vi "Console GUI (Read and Write).vi"() -> ()   [LabVIEW 2017, in "Communications Console Library.lvlib"]
uses:
  Communications Console Library.lvlib
  Typedefs/Console GUI-Program State--Enum.ctl
  <vilib>/event_ctls.llb/eventvkey.ctl
  Communications/Typedefs/Functional Global Variable Action--Enum.ctl
  Communications/Communications Library.lvlib
panel:
  out "Sending":bool
  out "Receiving":bool
  in  "User Input":string
  out "Console Text":string
  # "Command to Send"
  # ">"
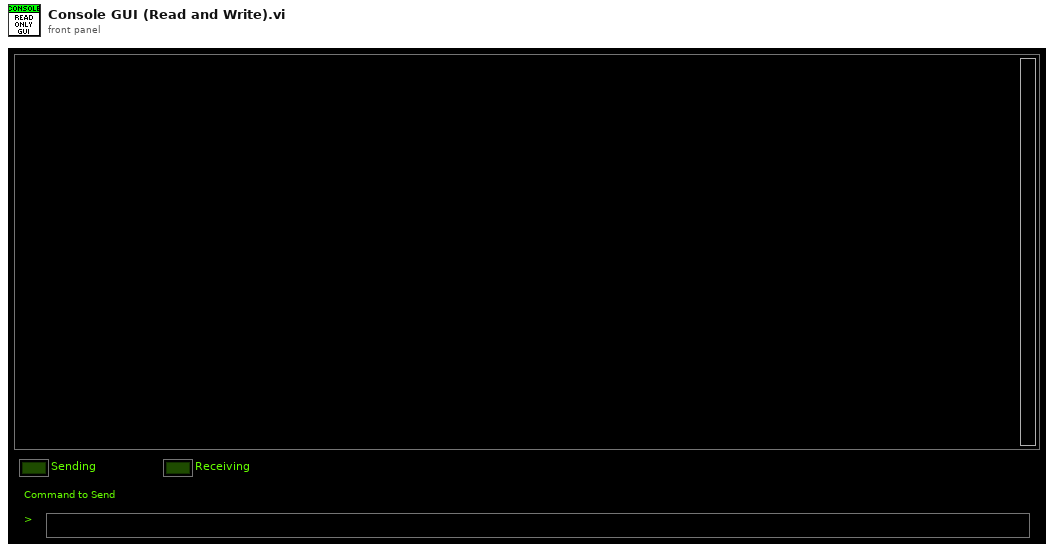
[diagram p1: front panel]
types:
  T1 = typedef "Communications Console Library.lvlib/Console GUI-Program State--Enum.ctl" = enum16{"Load Configuration", "Send Message", "Wait", "Update GUI", "Read TCP Log File"}
  T2 = typedef "eventvkey.ctl" = enum16{"ASCII", "Enter", "Return", "Shift", "Ctrl", "Alt", "Cmd", "Opt", "Caps", "NumLock", "Clear", "Break", "Up", "Down", "Left", "Right", "Insert", "Delete", "Home", "End", "PageUp", "PageDown", "Escape", "Help", "Pause", "ScrollLock", "F1", "F2", "F3", "F4", "F5", "F6", "F7", "F8", "F9", "F10", "F11", "F12", "F13", "F14", "F15", "F16", "F17", "F18", "F19", "F20", "F21", "F22", "F23", "F24", "Play", "VolumeUp", "VolumeDown", "Mute", "Two Byte Char"}
  T3 = typedef "Communications Library.lvlib/Functional Global Variable Action--Enum.ctl" = enum16{"Initialise", "Write Module Config", "Write Carrier Config", "Read"}
  T4 = typedef "Communications Library.lvlib/DTACQ Module Carrier Configuration--Cluster.ctl" = cluster{"Name":string, "IP":string, "Control Port":i32, "Timeout (ms)":i32, "Continuous Capture Port (Multiplexed)":i32, "Start HIL Shot Port":i32, "AWG Upload Port (Multiplexed)":i32, "Download Captured Data Port (Multiplexed)":i32, "Module Slots":i32, "Module Configurations":T5[]}
  T5 = typedef "Communications Library.lvlib/DTACQ Module Configuration--Cluster.ctl" = cluster{"Name":string, "Position":string, "Module Type":T6, "Control Port":i32, "Timeout (ms)":i32, "Channels":i32}
  T6 = typedef "Communications Library.lvlib/DTACQ Device Type--Enum.ctl" = enum16{"Carrier", "Analog In Module", "Analog Out Module", "Generic Module"}
  T7 = typedef "Communications Library.lvlib/DTACQ Connection Data--Cluster.ctl" = cluster{"Description":string, "Address":string, "Port":u16, "timeout (ms)":i32, "Termination Character":string, "TCP Connection Reference":refnum<k5>, "Open Connection":bool}
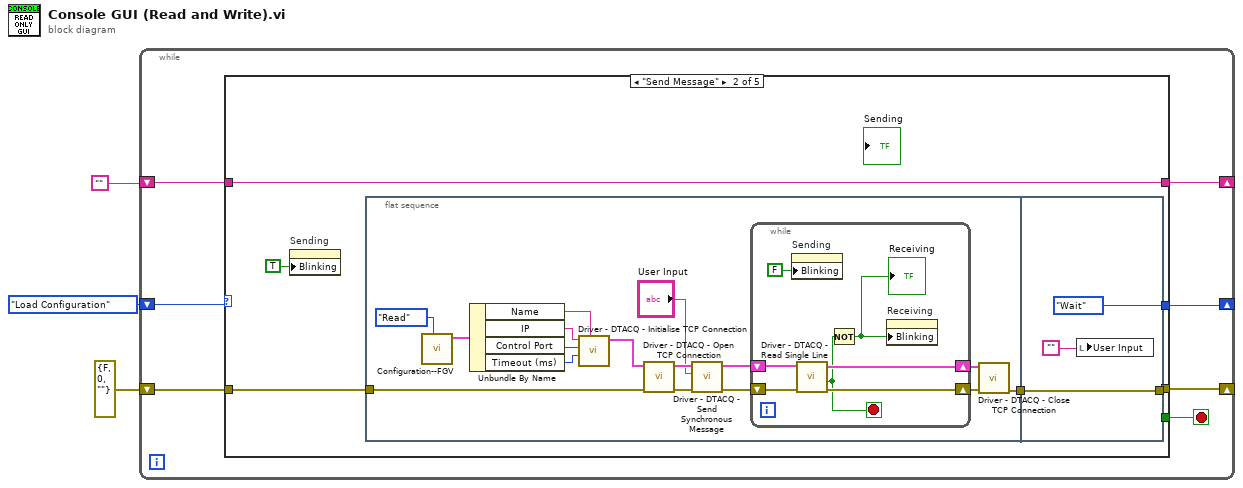
[diagram p0: block diagram]
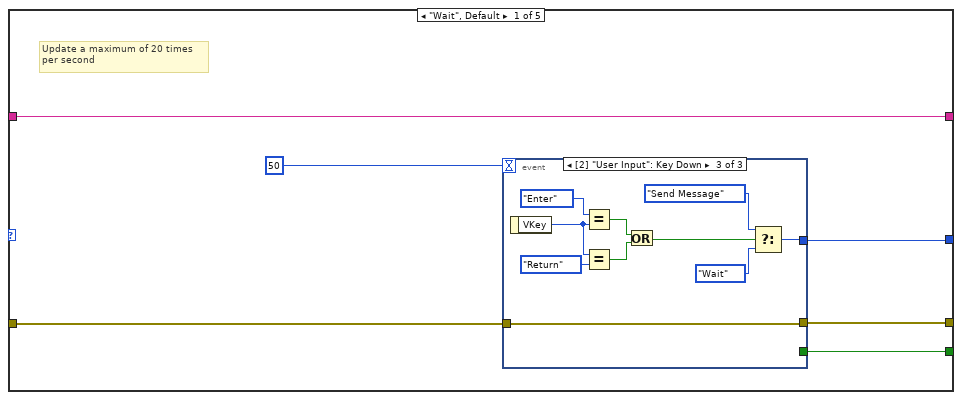
[diagram p2: hidden frame]
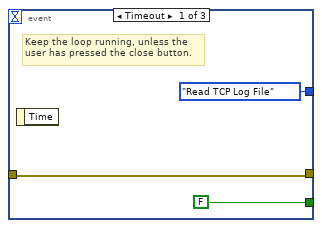
[diagram p3: hidden frame]
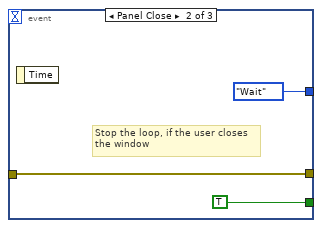
[diagram p4: hidden frame]
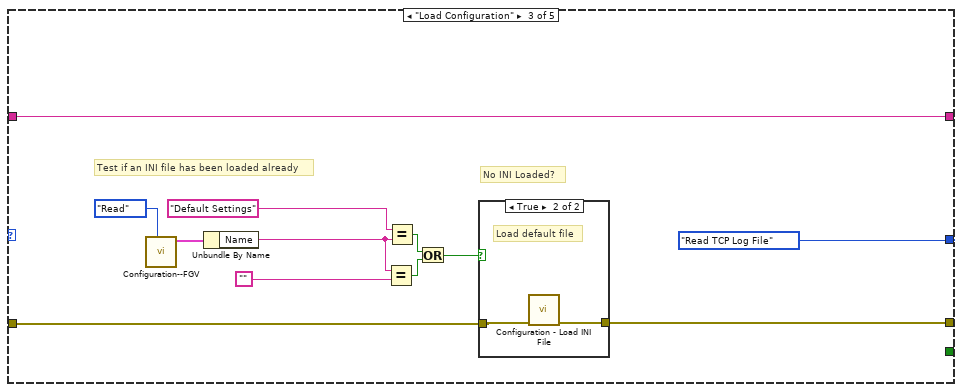
[diagram p5: hidden frame]
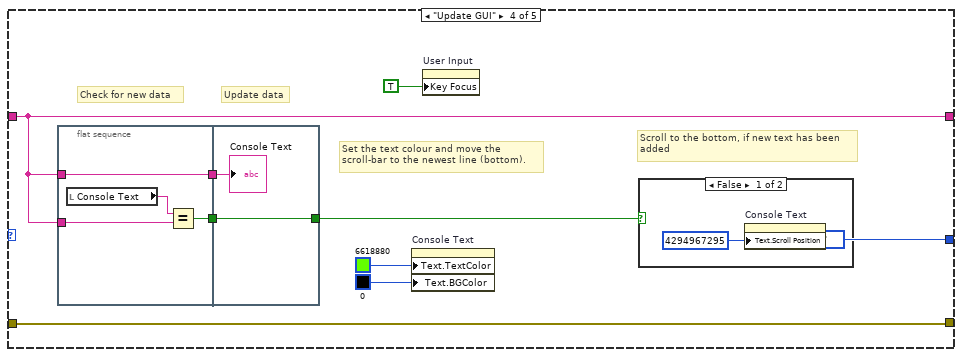
[diagram p7: hidden frame]
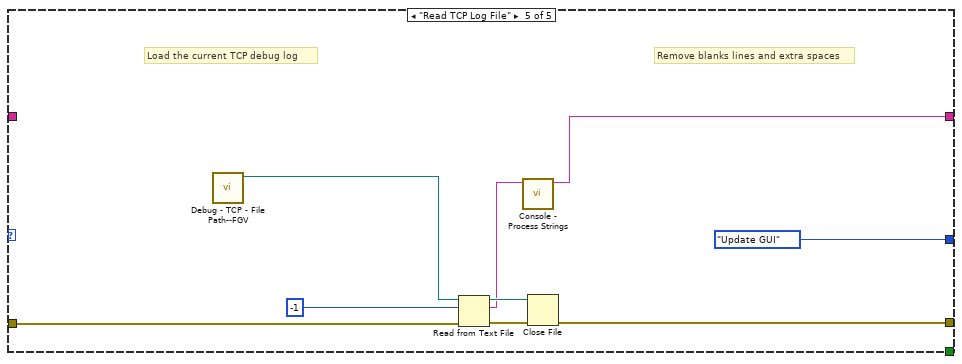
[diagram p9: hidden frame]
diagram:
  n1 = while {
    shift-right: [w10] -> _
    shift-left: "" -> [w9]
    shift-right: [w7] -> _
    shift-left: Console_GUI-Program_State--Enum."Load Configuration" ("Console GUI State") -> [w8]
    shift-right: [w5] -> _
    shift-left: errorcluster {"status"=FALSE, "code"=0, "source"=""} ("error out") -> [w6]
    stop <- w4 stop-if-true
    n2 = case shown="\"Send Message\"" w8 {
      tunnel: [w16 w38 w75 w80 w95] -> w10
      tunnel: w9 -> [w16 w38 w75 w80 _]
      tunnel: [w11 Console_GUI-Program_State--Enum."Wait" ("Console GUI State") Console_GUI-Program_State--Enum."Read TCP Log File" ("Console GUI State") Console_GUI-Program_State--Enum."Wait" ("Console GUI State") Console_GUI-Program_State--Enum."Update GUI" ("Console GUI State")] -> w7
      tunnel: w6 -> [w14 w36 w67 w84 w99]
      tunnel: [w13 w34 w66 w84 w98] -> w5
      tunnel: [w12 _ _ _ _] -> w4
      frame "Wait", Default {
        # "Update a maximum of 20 times\nper second"
        n3 = event shown="[2] \"User Input\": Key Down" {
          selector: _ -> [_ _ _]
          dyn-events: _ -> [_ _ _]
          timeout: 50 -> [_ _ _]
          tunnel: w14 -> [w19 w22 w27]
          tunnel: [w19 w22 w27] -> w13
          tunnel: [FALSE TRUE _] -> w12
          tunnel: [Console_GUI-Program_State--Enum."Read TCP Log File" ("Console GUI State") Console_GUI-Program_State--Enum."Wait" ("Console GUI State") w24] -> w11
          event Timeout {
            # "Keep the loop running, unless the\nuser has pressed the close button."
            n4 = event-data() -> ()  [unwired: 1 in, 1 out]
          }
          event Panel Close {
            # "Stop the loop, if the user closes\nthe window"
            n5 = event-data() -> ()  [unwired: 1 in, 1 out]
          }
          event "User Input": Key Down {
            n6 = event-data() -> ("VKey"=w30:T2)  [unwired: 1 in]
            n7 = Equal?(x=eventvkey."Enter" ("VKey"), y=w30) -> (x = y?=w28:bool)
            n8 = Equal?(x=w30, y=eventvkey."Return" ("VKey")) -> (x = y?=w29:bool)
            n9 = Or(x=w28, y=w29) -> (x .or. y?=w25:bool)
            n10 = Select(t=Console_GUI-Program_State--Enum."Send Message" ("Console GUI State"), s=w25, f=Console_GUI-Program_State--Enum."Wait") -> (s? t:f=w24:T1)
          }
        }
      }
      frame "Send Message" {
        n11 = property on="Sending" class="Bool (strict)"("Blinking"=TRUE) -> ()  [unwired: 2 in, 2 out]
        n12 = flat-sequence {
          tunnel: w36 -> [w48]
          tunnel: [w47] -> w35
          tunnel: [w62] -> w34
          tunnel: w35 -> [w62]
          frame #0 {
            n13 = call "Configuration--FGV.vi"("Functional Global Action"=Functional_Global_Variable_Action--Enum."Read") -> ("Carrier Configuration Out"=w46:T4)  [unwired: 9 in, 1 out]
            n14 = Unbundle By Name(w46) -> ("Name"=w52:string, "IP"=w51:string, "Control Port"=w50:i32, "Timeout (ms)"=w49:i32)
            n15 = call "Driver - DTACQ - Initialise TCP Connection.vi"("Description"=w52, "timeout (ms)"=w49, "Port"=w50, "Address"=w51) -> ("DTACQ Connection Data Out"=w53:T7)  [unwired: 7 in]
            n16 = call "Driver - DTACQ - Open TCP Connection.vi"("error in"=w48, "DTACQ Connection Data In"=w53) -> ("error out"=w45:errorcluster, "DTACQ Connection Data Out"=w44:T7)  [unwired: 8 in]
            n17 = call "Driver - DTACQ - Send Synchronous Message.vi"("error in"=w45, "Message to Send"="User Input", "DTACQ Connection Data In"=w44) -> ("error out"=w42:errorcluster, "DTACQ Connection Data Out"=w43:T7)  [unwired: 5 in, 2 out]
            n18 = while {
              shift-right: [w58] -> w40
              shift-left: w43 -> [w61]
              shift-right: [w59] -> w41
              shift-left: w42 -> [w60]
              stop <- w57 stop-if-true
              n19 = property on="Sending" class="Bool (strict)"("Blinking"=FALSE) -> ()  [unwired: 2 in, 2 out]
              n20 = call "Driver - DTACQ - Read Single Line.vi"("error in"=w60, "DTACQ Connection Data In"=w61) -> ("error out"=w59:errorcluster, "Timed Out"=w57:bool, "DTACQ Connection Data Out"=w58:T7)  [unwired: 6 in, 1 out]
              n21 = Not(x=w57) -> (.not. x?=w56:bool)
              "Receiving" <- w56
              n22 = property on="Receiving" class="Bool (strict)"("Blinking"=w56) -> ()  [unwired: 2 in, 2 out]
            }
            n23 = call "Driver - DTACQ - Close TCP Connection.vi"("error in"=w41, "DTACQ Connection Data In"=w40) -> ("error out"=w47:errorcluster)  [unwired: 8 in, 1 out]
          }
          frame #1 {
            n24 = local write "User Input"("") -> ()
          }
        }
      }
      frame "Load Configuration" {
        # "No INI Loaded?"
        # "Test if an INI file has been loaded already"
        n25 = call "Configuration--FGV.vi"("Functional Global Action"=Functional_Global_Variable_Action--Enum."Read") -> ("Carrier Configuration Out"=w73:T4)  [unwired: 9 in, 1 out]
        n26 = Unbundle By Name(w73) -> ("Name"=w72:string)
        n27 = Equal?(x=w72, y="") -> (x = y?=w69:bool)
        n28 = Equal?(x="Default Settings" ("Name"), y=w72) -> (x = y?=w68:bool)
        n29 = Or(x=w68, y=w69) -> (x .or. y?=w65:bool)
        n30 = case shown="True" w65 {
          tunnel: w67 -> [w76 w78]
          tunnel: [w76 w77] -> w66
          frame False {
            # "INI already loaded,\ndo nothing."
          }
          frame True {
            # "Load default file"
            n31 = call "Configuration - Load INI File.vi"("error in"=w78) -> ("error out"=w77:errorcluster)  [unwired: 9 in, 1 out]
          }
        }
      }
      frame "Update GUI" {
        # "Check for new data"
        # "Scroll to the bottom, if new text has been\nadded"
        # "Update data"
        # "Set the text colour and move the \nscroll-bar to the newest line (bottom)."
        n32 = flat-sequence {
          tunnel: w80 -> [w91]
          tunnel: [w89] -> w82
          tunnel: w80 -> [w88]
          tunnel: [w88] -> w81
          tunnel: [w93] -> w79
          tunnel: w82 -> [w93]
          tunnel: w81 -> [w92]
          frame #0 {
            n33 = local read "Console Text"() -> (w90:string)
            n34 = Equal?(x=w90, y=w91) -> (x = y?=w89:bool)
          }
          frame #1 {
            "Console Text" <- w92
          }
        }
        n35 = property on="Console Text" class="Str"("Text.TextColor"=u32 6618880, "Text.BGColor"=u32 0) -> ()  [unwired: 2 in, 2 out]
        n36 = property on="User Input" class="Str"("Key Focus"=TRUE) -> ()  [unwired: 2 in, 2 out]
        n37 = case shown="False" w79 {
          frame False {
            n38 = property on="Console Text" class="Str"("Text.Scroll Position"=u32 4294967295) -> ()  [unwired: 2 in, 2 out]
          }
          frame True {
          }
        }
      }
      frame "Read TCP Log File" {
        # "Remove blanks lines and extra spaces"
        # "Load the current TCP debug log"
        n39 = call "Debug - TCP - File Path--FGV.vi"() -> ("Debug Pathname"=w96:path)  [unwired: 11 in]
        n40 = Read from Text File(file (use dialog)=w96, count=-1, error in=w99) -> (refnum out=w102:refnum<file>, text=w100:string, error out=w101:errorcluster)  [unwired: 1 in, 1 out]
        n41 = call "Console - Process Strings.vi"("Unprocessed String"=w100) -> ("Processed String"=w95:string)  [unwired: 10 in]
        n42 = Close File(refnum=w102, error in=w101) -> (error out=w98:errorcluster)  [unwired: 1 out]
      }
    }
  }
